vi "Read image from usb.vi"() -> ()   [LabVIEW 2018]
uses:
  <vilib>/vision/driver/Vision Acquisition Express Utility VIs.llb/Vision Acquisition Path Convert (Path).vi
panel:
  out "Image Out":T1(plugin-control)
  in  "error in":errorcluster
  out "error out":errorcluster
  in  "stop":bool
  in  "logfile base name 2":string="logfile"
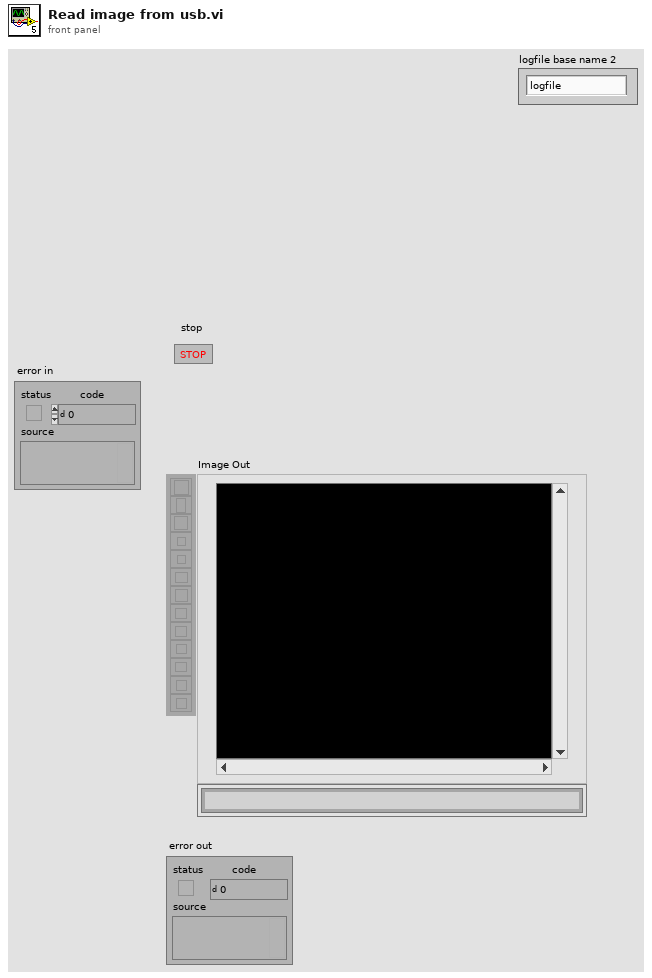
[diagram p1: front panel]
types:
  T1 = typedef "IMAQ Image.ctl" = refnum<image>
  T2 = typedef "Image Type" = u32
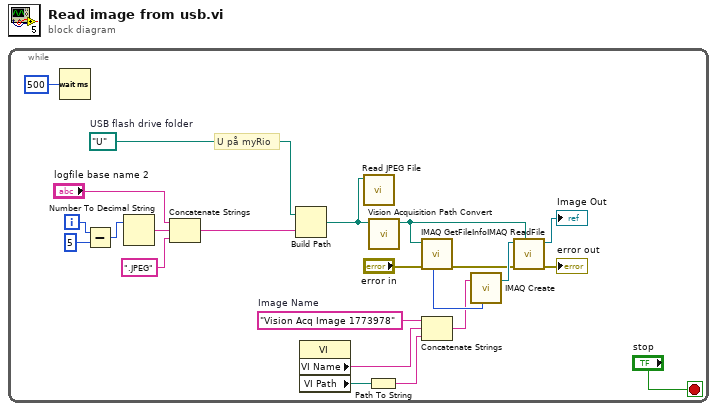
[diagram p0: block diagram]
diagram:
  n1 = while {
    i -> [w17]
    stop <- "stop" stop-if-true
    w5 = "Vision Acq Image 1773978"  # Image Name
    w22 = path "U:/"  # USB flash drive folder
    # "U på myRio"
    n2 = Wait (ms)(milliseconds to wait=u32 500) -> ()  [unwired: 1 out]
    n3 = Subtract(x=w17, y=5) -> (x-y=w23:i32)
    n4 = Number To Decimal String(number=w23) -> (decimal integer string=w18:string)  [unwired: 1 in]
    n5 = Concatenate Strings "Concatenate Strings"("logfile base name 2", w18, ".JPEG" ("string")) -> (w20:string)
    n6 = Build Path(base path=w22, name or relative path=w20) -> (appended path=w1:path)
    n7 = property class="VI"() -> ("VI Name"=w7:string, "VI Path"=w8:path)  [unwired: 2 in, 2 out]
    n8 = call <vilib>:"Read JPEG File.vi"("path to JPEG file"=w1) -> ()  [unwired: 8 in, 3 out]
    n9 = Path To String(path=w8) -> (string=w6:string)
    n10 = call-poly <vilib>:"Vision Acquisition Path Convert.vi"("Path In"=w1) -> ("Path Out"=w2:path)  [unwired: 10 in]
    n11 = call "IMAQ GetFileInfo"("error in (no error)"="error in", "File Path"=w2) -> ("error out"=w9:errorcluster, "Image Type"=w11:T2)  [unwired: 8 out]
    n12 = Concatenate Strings(w5, w7, w6) -> (w4:string)
    n13 = call "IMAQ Create"("Image Name"=w4, "Image Type"=w11) -> ("New Image"=w13:T1)  [unwired: 2 in, 2 out]
    n14 = call "IMAQ ReadFile"("File Path"=w2, "error in (no error)"=w9, "Image"=w13) -> ("error out"=→"error out":errorcluster, "Image Out"=→"Image Out":T1)  [unwired: 2 in, 5 out]
  }
